vi "Destroy.vi"(8 "error in (no error)":errorcluster, 11 "FINE SIM Motion Axis in":refnum<class "FINE SIM Motion Axis.lvclass">) -> (0 "error out":errorcluster, 3 "FINE SIM Motion Axis out":refnum<class "FINE SIM Motion Axis.lvclass">)   [LabVIEW 2022 SP3, in "FINE SIM Motion Axis.lvclass"]
uses:
  FINE SIM Motion Axis.lvclass
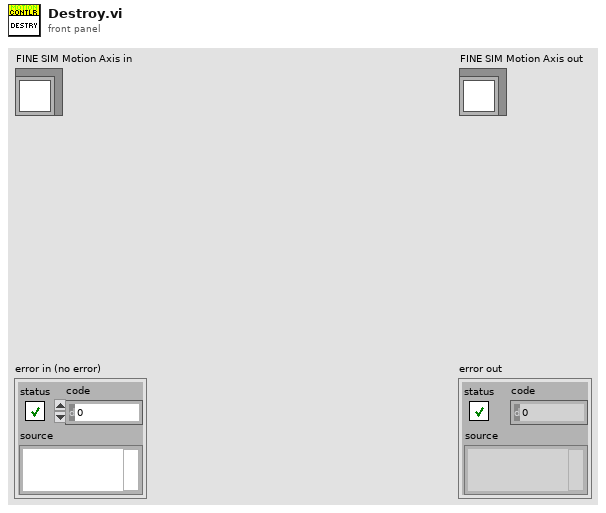
[diagram p1: front panel]
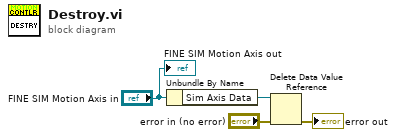
[diagram p0: block diagram]
diagram:
  n1 = Unbundle By Name("FINE SIM Motion Axis in") -> ("Sim Axis Data"=w3:refnum<data-value>)
  n2 = Delete Data Value Reference(data value reference=w3, error in="error in (no error)") -> (error out=→"error out":errorcluster)  [unwired: 1 out]
  "FINE SIM Motion Axis out" <- "FINE SIM Motion Axis in"
